vi "Write_File_Simple.vi"(2 "append to file? (new file:F)":bool, 3 "character string":string, 4 "file path":path) -> (0 "error out":errorcluster, 1 "file path Out":path)   [LabVIEW 2010]
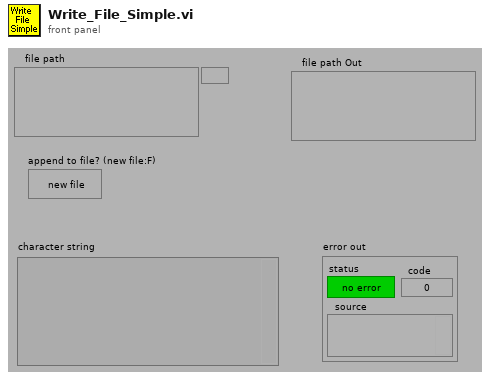
[diagram p1: front panel]
types:
  T1 = enum16{"deny read/write", "deny write-only", "deny none"}
  T2 = enum16{"read/write", "read-only", "write-only", "write-only (truncate)"}
  T3 = enum16{"open", "replace", "create", "open or create", "replace or create", "replace or create with confirmation"}
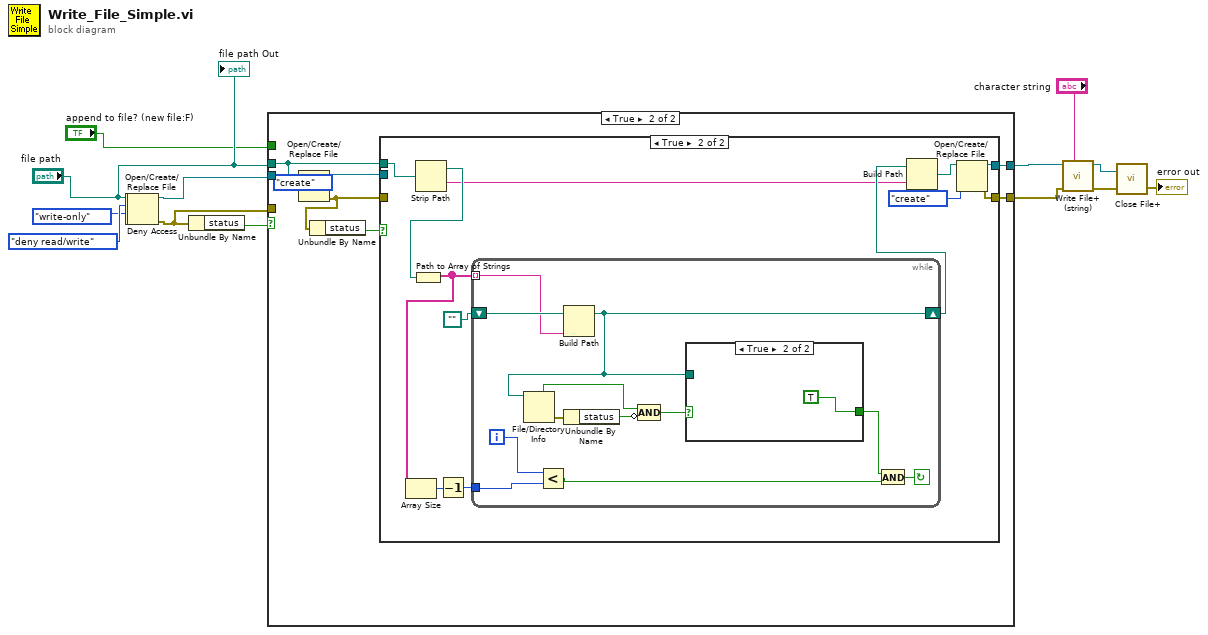
[diagram p0: block diagram]
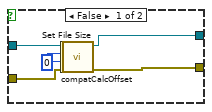
[diagram p3: hidden frame]
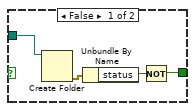
[diagram p5: hidden frame]
diagram:
  n1 = Open/Create/Replace File(file path (use dialog)="file path", access (0:read/write)=T2."write-only" ("open mode (0)")) -> (refnum out=w1:refnum<file>, error out=w2:errorcluster)  [unwired: 1 in, 4 out]
  n2 = Deny Access(4:w2, 6:T1."deny read/write" ("deny mode (2)"), 7:w1) -> (0:w5:errorcluster, 3:w11:refnum<file>)
  n3 = Unbundle By Name(w5) -> ("status"=w13:bool)
  n4 = case shown="True" w13 {
    tunnel: "file path" -> [_ w34]
    tunnel: w11 -> [w20 _]
    tunnel: [w19 w37] -> w10
    tunnel: [w18 w36] -> w9
    tunnel: w5 -> [w17 _]
    tunnel: "append to file? (new file:F)" -> [w16 _]
    frame False {
      n5 = case shown="True" w16 {
        tunnel: w20 -> [w27 w29]
        tunnel: [w26 w29] -> w19
        tunnel: [w25 w30] -> w18
        tunnel: w17 -> [w24 w30]
        frame False {
          w28 = 0
          n6 = call <vilib>:"compatCalcOffset.vi"("error in"=w24, "pos offset (0)"=w28, "pos mode (0:1)"=w28, "refnum"=w27) -> ("error out"=w23:errorcluster, "offset"=w22:i32, "dup refnum"=w21:refnum<file>)  [unwired: 5 out]
          n7 = Set File Size(4:w23, 6:w22, 7:w21) -> (0:w25:errorcluster, 3:w26:refnum<file>)
        }
        frame True {
        }
      }
    }
    frame True {
      n8 = Open/Create/Replace File(file path (use dialog)=w34, operation (0:open)=T3."create") -> (refnum out=w33:refnum<file>, error out=w32:errorcluster)  [unwired: 1 in, 4 out]
      n9 = Unbundle By Name(w32) -> ("status"=w35:bool)
      n10 = case shown="True" w35 {
        tunnel: w34 -> [_ w45]
        tunnel: [w39 w48] -> w37
        tunnel: [w38 w47] -> w36
        tunnel: w33 -> [w39 _]
        tunnel: w32 -> [w38 _]
        frame False {
        }
        frame True {
          n11 = Strip Path(path=w45) -> (stripped path=w44:path, name=w42:string)
          n12 = Path to Array of Strings(0:w44) -> (2:w50:string[])  [unwired: 1 out]
          n13 = Array Size(array=w50) -> (size(s)=w51:i32)
          n14 = Decrement(x=w51) -> (x-1=w49:i32)
          n15 = while {
            tunnel: w49 -> [w60]
            shift-left: path "" ("appended path") -> [w63]
            shift-right: [w56] -> w43
            tunnel: w50 -> [w62] mode=indexing
            i -> [w61]
            stop <- w58 continue-if-true
            n16 = Less?(x=w61, y=w60) -> (x < y?=w59:bool)
            n17 = Build Path(base path=w63, name or relative path=w62) -> (appended path=w56:path)
            n18 = File/Directory Info(path=w56) -> (directory=w53:bool, error out=w55:errorcluster)  [unwired: 1 in, 5 out]
            n19 = Unbundle By Name(w55) -> ("status"=w54:bool)
            n20 = Compound Arithmetic op=AND(w53, invert w54) -> (w52:bool)
            n21 = case shown="True" w52 {
              tunnel: w56 -> [w67 _]
              tunnel: [w64 TRUE] -> w57
              frame False {
                n22 = Create Folder(path (use dialog)=w67) -> (error out=w66:errorcluster)  [unwired: 1 in, 3 out]
                n23 = Unbundle By Name(w66) -> ("status"=w65:bool)
                n24 = Not(x=w65) -> (.not. x?=w64:bool)
              }
              frame True {
              }
            }
            n25 = And(x=w57, y=w59) -> (x .and. y?=w58:bool)
          }
          n26 = Build Path(base path=w43, name or relative path=w42) -> (appended path=w41:path)
          n27 = Open/Create/Replace File(file path (use dialog)=w41, operation (0:open)=T3."create") -> (refnum out=w48:refnum<file>, error out=w47:errorcluster)  [unwired: 1 in, 4 out]
        }
      }
    }
  }
  n28 = call <vilib>:"Write File+ (string).vi"("string"="character string", "error in (no error)"=w9, "refnum"=w10) -> ("error out"=w8:errorcluster, "dup refnum"=w7:refnum<file>)  [unwired: 2 in, 3 out]
  n29 = call <vilib>:"Close File+.vi"("error in (no error)"=w8, "refnum"=w7) -> ("error out"=→"error out":errorcluster)  [unwired: 5 out]
  "file path Out" <- "file path"
